vi "InitBGImages.vi"() -> (3 "BGImages":T1)   [LabVIEW 2013, in "MagAnalysis_Online.lvclass"]
uses:
  MagAnalysis_Online.lvclass
  bgImages_tyudef.ctl
  <vilib>/vision/Image Controls.llb/IMAQ Image.ctl
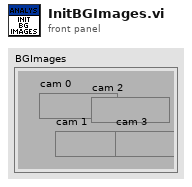
[diagram p1: front panel]
types:
  T1 = typedef "bgImages_tyudef.ctl" = cluster{"cam 0":T2, "cam 1":T2, "cam 2":T2, "cam 3":T2}
  T2 = typedef "IMAQ Image.ctl" = refnum<image>
  T3 = typedef "Image Type" = u32
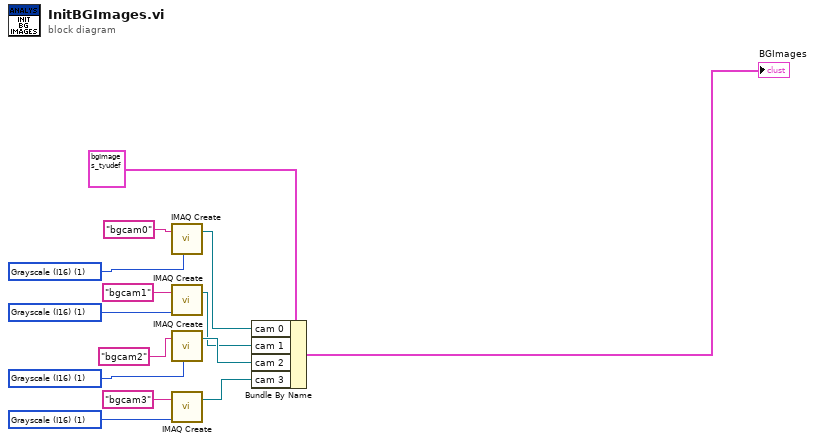
[diagram p0: block diagram]
diagram:
  w7 = T3 1 items=["Grayscale (U8)", "Grayscale (I16)", "Grayscale (SGL)", "Complex (CSG)", "RGB (U32)", "HSL (U32)", "RGB (U64)", "Grayscale (U16)"] ("Image Type")
  w6 = T3 1 items=["Grayscale (U8)", "Grayscale (I16)", "Grayscale (SGL)", "Complex (CSG)", "RGB (U32)", "HSL (U32)", "RGB (U64)", "Grayscale (U16)"] ("Image Type")
  w2 = T3 1 items=["Grayscale (U8)", "Grayscale (I16)", "Grayscale (SGL)", "Complex (CSG)", "RGB (U32)", "HSL (U32)", "RGB (U64)", "Grayscale (U16)"] ("Image Type")
  w3 = T3 1 items=["Grayscale (U8)", "Grayscale (I16)", "Grayscale (SGL)", "Complex (CSG)", "RGB (U32)", "HSL (U32)", "RGB (U64)", "Grayscale (U16)"] ("Image Type")
  n1 = call "IMAQ Create"("Image Name"="bgcam0", "Image Type"=w3) -> ("New Image"=w10:T2)  [unwired: 3 in, 1 out]
  n2 = call "IMAQ Create"("Image Name"="bgcam1", "Image Type"=w2) -> ("New Image"=w11:T2)  [unwired: 3 in, 1 out]
  n3 = call "IMAQ Create"("Image Name"="bgcam2", "Image Type"=w6) -> ("New Image"=w12:T2)  [unwired: 3 in, 1 out]
  n4 = call "IMAQ Create"("Image Name"="bgcam3", "Image Type"=w7) -> ("New Image"=w13:T2)  [unwired: 3 in, 1 out]
  n5 = Bundle By Name(cluster=T1 {"cam 0"=refnum, "cam 1"=refnum, "cam 2"=refnum, "cam 3"=refnum} ("BGImages"), "cam 0"=w10, "cam 1"=w11, "cam 2"=w12, "cam 3"=w13) -> (→"BGImages":T1)
